vi "CallCommunicate.vi"(8 "error in (no error)":errorcluster, 11 "Sender in":refnum<class "Sender.lvclass">) -> (0 "error out":errorcluster, 2 "Communication.lvclass":refnum<class "Communication.lvclass">, 3 "Sender out":refnum<class "Sender.lvclass">)   [LabVIEW 2023, in "Sender.lvclass"]
doc: "Sends the data from the sender class to the communicate class."
uses:
  Sender.lvclass
  Communication/Communication.lvclass
  Sender.lvclass/Sender.ctl
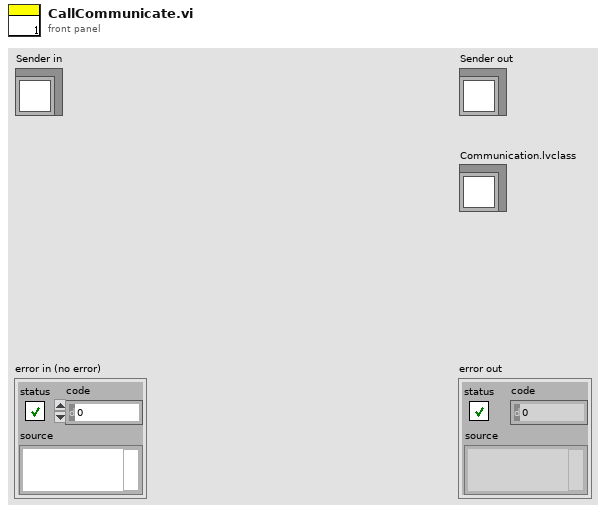
[diagram p1: front panel]
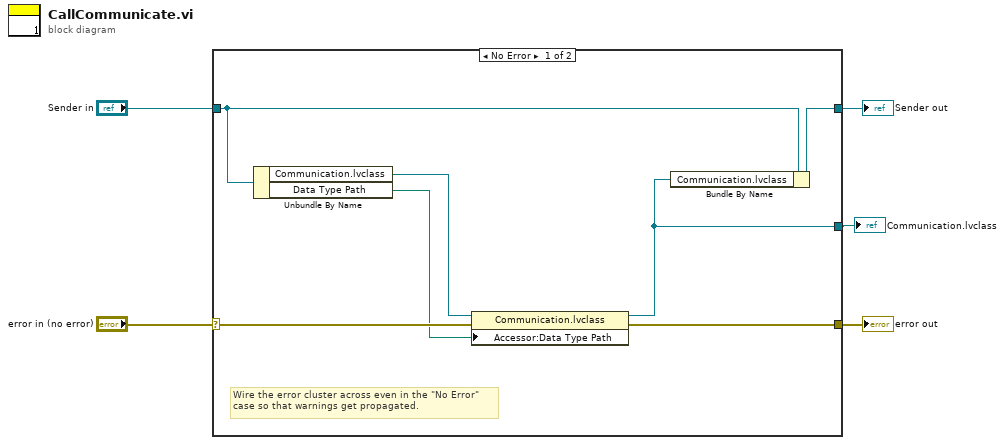
[diagram p0: block diagram]
diagram:
  n1 = case shown="No Error" "error in (no error)" {
    selector: "error in (no error)" -> [w12 w14]
    tunnel: [w11 w14] -> w4
    tunnel: [w9 w13] -> w2
    tunnel: "Sender in" -> [w7 w13]
    tunnel: [w8 _] -> w1
    frame No Error {
      # "Wire the error cluster across even in the \"No Error\"\ncase so that warnings get propagated."
      n2 = Unbundle By Name(w7) -> ("Communication.lvclass"=w10:refnum<class "Communication.lvclass">, "Data Type Path"=w6:path)
      n3 = property class="Communication.lvclass"(reference=w10, error in=w12, "Accessor:Data Type Path"=w6) -> (reference out=w8:refnum<class "Communication.lvclass">, error out=w11:errorcluster)
      n4 = Bundle By Name(cluster=w7, "Communication.lvclass"=w8) -> (w9:refnum<class "Sender.lvclass">)
    }
    frame Error {
    }
  }
  "error out" <- w4
  "Sender out" <- w2
  "Communication.lvclass" <- w1
